vi "Logging Message Loop.vi"(8 "error in (no error)":cluster{"状态":bool, "代码":i32, "源":string} caption="错误输入（无错误）", 10 "数据队列":refnum<queue>, 11 "消息队列":T1) -> (0 "error out":cluster{"状态":bool, "代码":i32, "源":string} caption="错误输出")   [LabVIEW 2018, in "Logging.lvlib"]
doc: "消息循环子VI负责处理与记录数据相关的消息。"
uses:
  Logging.lvlib
  support/Message Queue/All Message Queues.ctl
  support/Message Queue/Message Cluster.ctl
  Logging Configuration.ctl
  Logging State.ctl
  support/Message Queue/Enqueue Message (Single).vi
  <vilib>/Utility/error.llb/Error Cluster From Error Code.vi
  <vilib>/ErrorRing/Error Ring.xnode
  support/Message Queue/Message Queue.lvlib
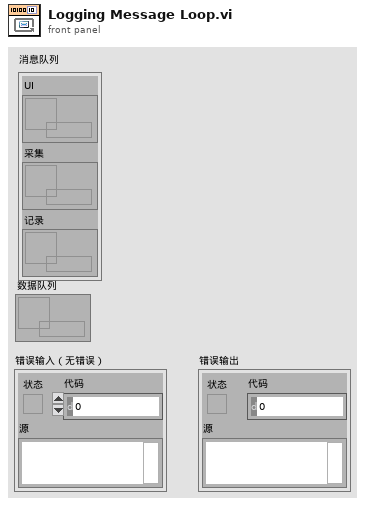
[diagram p1: front panel]
types:
  T1 = typedef "Message Queue.lvlib/All Message Queues.ctl" = cluster{"UI":refnum<queue>, "采集":refnum<queue>, "记录":refnum<queue>}
  T2 = typedef "Logging.lvlib/Logging Configuration.ctl" = cluster{"记录文件基路径":path, "TDMS文件引用":refnum<k34>}
  T3 = typedef "Logging.lvlib/Logging State.ctl" = enum16{"Idle", "Logging"}
  T4 = enum16{"open", "open or create", "create or replace", "create", "open (read-only)"}
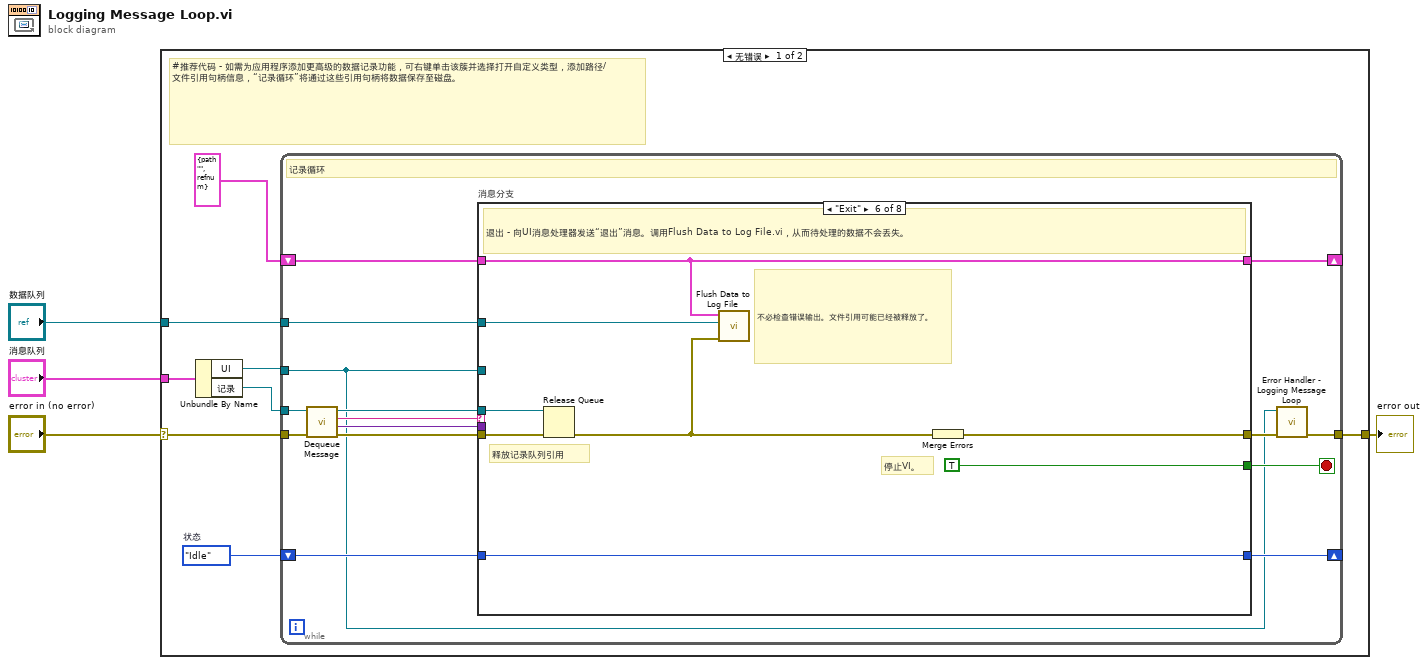
[diagram p0: block diagram]
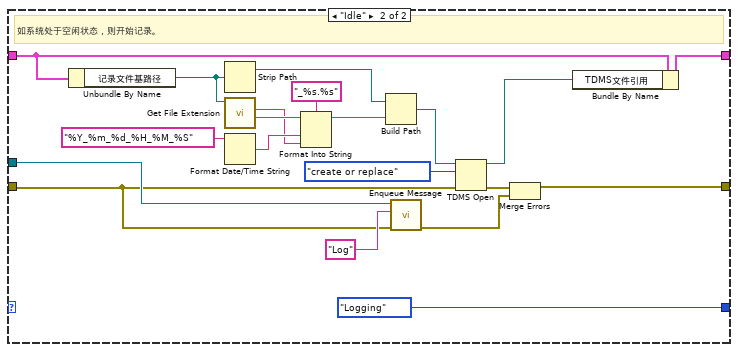
[diagram p4: hidden frame]
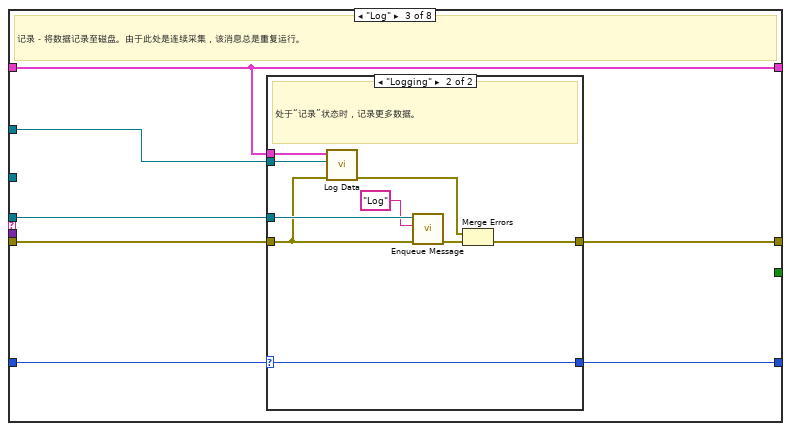
[diagram p5: hidden frame]
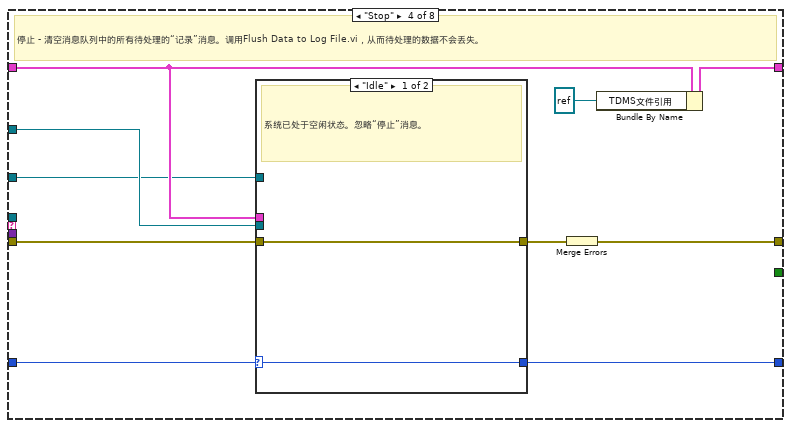
[diagram p7: hidden frame]
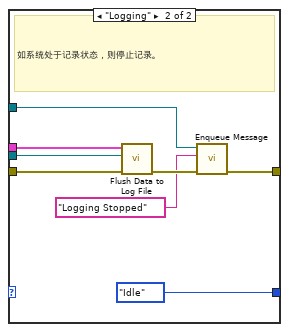
[diagram p8: hidden frame]
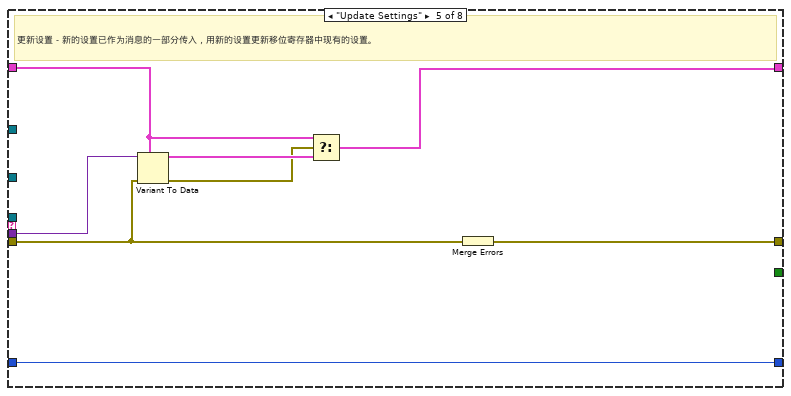
[diagram p9: hidden frame]
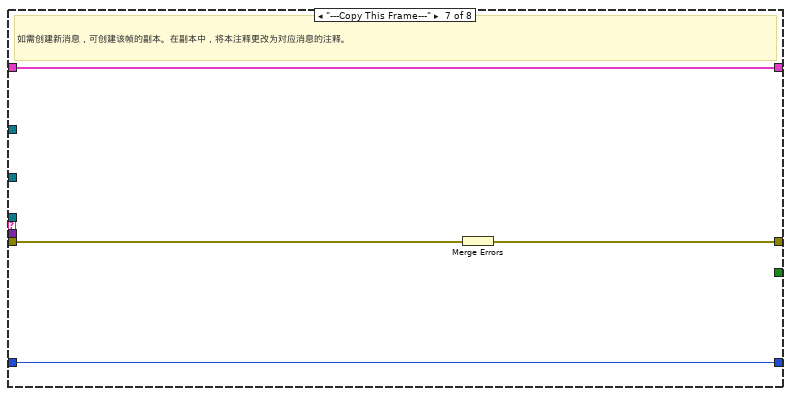
[diagram p10: hidden frame]
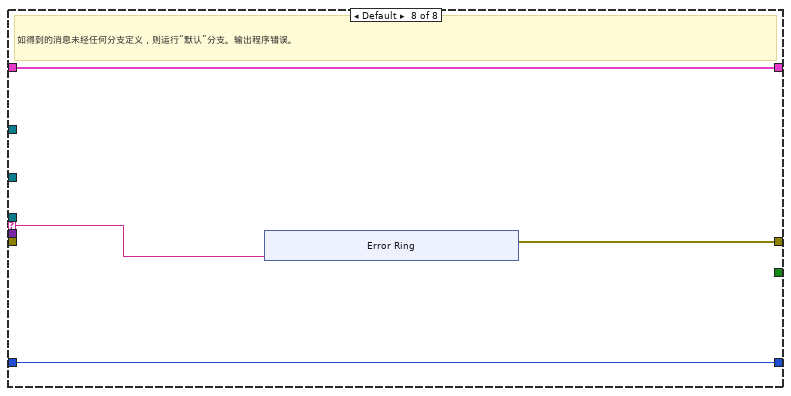
[diagram p11: hidden frame]
diagram:
  n1 = case shown="无错误" "error in (no error)" {
    selector: "error in (no error)" -> [w8 w130]
    tunnel: "消息队列" -> [w12 _]
    tunnel: [w10 w130] -> w3
    tunnel: "数据队列" -> [w7 _]
    frame No Error {
      w5 = Logging_State."Idle"  # 状态
      # "#推荐代码 - 如需为应用程序添加更高级的数据记录功能，可右键单击该簇并选择打开自定义类型，添加路径/文件引用句柄信息，“记录循环”将通过这些引用句柄将数据保存至磁盘。"
      n2 = Unbundle By Name(w12) -> ("UI"=w6:refnum<queue>, "记录"=w11:refnum<queue>)
      n3 = while {
        tunnel: w11 -> [w19]
        shift-right: [w26] -> _
        shift-left: T2 {"记录文件基路径"=path "", "TDMS文件引用"=refnum} ("Logging Configuration") -> [w27]
        tunnel: w6 -> [w13]
        tunnel: w7 -> [w18]
        shift-right: [w16] -> _
        shift-left: w5 -> [w17]
        tunnel: w8 -> [w24]
        tunnel: [w15] -> w10
        stop <- w25 stop-if-true
        # "记录循环"
        n4 = call "Dequeue Message.vi"("error in (no error)"=w24, "消息队列"=w19) -> ("error out"=w23:cluster{"状态":bool, "代码":i32, "源":string}, "消息数据"=w21:variant, "消息"=w22:string, "消息队列副本"=w20:refnum<queue>)  [unwired: 6 in]
        n5 = case "消息分支" shown="\"Exit\"" w22 {
          selector: w22 -> [_ _ _ _ _ _ _ w119]
          tunnel: w20 -> [_ w36 w66 _ _ w111 _ _]
          tunnel: w23 -> [w29 w35 w64 w82 w100 w112 w118 _]
          tunnel: [w29 w37 w67 w88 w106 w113 w116 w120] -> w14
          tunnel: w27 -> [w30 w34 w63 w83 w104 w109 w117 w122]
          tunnel: [w30 w33 w63 w86 w101 w109 w117 w122] -> w26
          tunnel: [_ _ _ _ _ TRUE _ _] -> w25
          tunnel: w21 -> [_ _ _ _ w105 _ _ _]
          tunnel: w13 -> [_ _ _ w79 _ _ _ _]
          tunnel: w18 -> [_ _ w65 w84 _ w108 _ _]
          tunnel: w17 -> [w28 w32 w62 w81 w99 w107 w115 w121]
          tunnel: [w28 w31 w61 w80 w99 w107 w115 w121] -> w16
          frame "Initialize" {
            # "初始化－第一次启动时将被调用。当前不包含任何操作。"
          }
          frame "Start" {
            # "开始 - 发送“记录”消息，开始记录。根据记录文件基路径的值生成一个唯一的带时间标识的TDMS文件名。"
            n6 = case shown="\"Logging\"" w32 {
              selector: w32 -> [w39 _]
              tunnel: [w38 w42] -> w37
              tunnel: w36 -> [_ w43]
              tunnel: w35 -> [w38 w41]
              tunnel: w34 -> [w40 w44]
              tunnel: [w40 w46] -> w33
              tunnel: [w39 Logging_State."Logging" ("State")] -> w31
              frame "Logging" {
                # "系统已处于记录状态。忽略“开始”消息。"
              }
              frame "Idle" {
                # "如系统处于空闲状态，则开始记录。"
                n7 = Unbundle By Name(w44) -> ("记录文件基路径"=w59:path)
                n8 = Strip Path(path=w59) -> (stripped path=w56:path)  [unwired: 1 out]
                n9 = call <vilib>:"Get File Extension.vi"("file"=w59) -> ("filename without extension"=w57:string, "lowercase file extension"=w53:string)  [unwired: 6 in, 3 out]
                n10 = Format Date/Time String(time format string (%c)="%Y_%m_%d_%H_%M_%S") -> (date/time string=w54:string)  [unwired: 2 in]
                n11 = Format Into String(format string="_%s.%s", initial string=w57, w54, w53) -> (resulting string=w52:string)  [unwired: 1 in, 1 out]
                n12 = Build Path(base path=w56, name or relative path=w52) -> (appended path=w51:path)
                n13 = call-poly "Enqueue Message.vi"("error in (no error)"=w41, "消息"="Log" ("Message"), "消息队列"=w43) -> ("error out"=w49:cluster{"状态":bool, "代码":i32, "源":string})  [unwired: 7 in, 1 out]
                n14 = TDMS Open(8:w41, 10:T4."create or replace" ("operation (0:open)"), 11:w51) -> (0:w50:errorcluster, 3:w47:refnum<k34>)  [unwired: 4 in]
                n15 = Merge Errors(w50, w49) -> (w42:errorcluster)
                n16 = Bundle By Name(cluster=w44, "TDMS文件引用"=w47) -> (w46:T2)
              }
            }
          }
          frame "Log" {
            # "记录－将数据记录至磁盘。由于此处是连续采集，该消息总是重复运行。"
            n17 = case shown="\"Logging\"" w62 {
              selector: w62 -> [w69 w71]
              tunnel: [w68 w78] -> w67
              tunnel: w66 -> [_ w76]
              tunnel: w65 -> [_ w75]
              tunnel: w64 -> [w68 w70]
              tunnel: w63 -> [_ w72]
              tunnel: [w69 w71] -> w61
              frame "Idle" {
                # "如记录处于空闲状态，则忽略“记录”消息。"
              }
              frame "Logging" {
                # "处于“记录”状态时，记录更多数据。"
                n18 = call "Log Data.vi"("error in (no error)"=w70, "数据队列"=w75, "记录配置"=w72) -> ("error out"=w74:cluster{"状态":bool, "代码":i32, "源":string})  [unwired: 8 in]
                n19 = call-poly "Enqueue Message.vi"("error in (no error)"=w70, "消息"="Log" ("Message"), "消息队列"=w76) -> ("error out"=w77:cluster{"状态":bool, "代码":i32, "源":string})  [unwired: 7 in, 1 out]
                n20 = Merge Errors(w74, w77) -> (w78:errorcluster)
              }
            }
          }
          frame "Stop" {
            # "停止 - 清空消息队列中的所有待处理的“记录”消息。调用Flush Data to Log File.vi，从而待处理的数据不会丢失。"
            n21 = case shown="\"Idle\"" w81 {
              selector: w81 -> [w89 _]
              tunnel: [w90 w93] -> w87
              tunnel: w84 -> [_ w97]
              tunnel: w83 -> [_ w96]
              tunnel: w82 -> [w90 w95]
              tunnel: [w89 Logging_State."Idle" ("State")] -> w80
              tunnel: w79 -> [_ w92]
              frame "Idle" {
                # "系统已处于空闲状态。忽略“停止”消息。"
              }
              frame "Logging" {
                # "如系统处于记录状态，则停止记录。"
                n22 = call "Flush Data to Log File.vi"("error in (no error)"=w95, "数据队列"=w97, "记录配置"=w96) -> ("error out"=w98:cluster{"状态":bool, "代码":i32, "源":string})  [unwired: 8 in]
                n23 = call-poly "Enqueue Message.vi"("error in (no error)"=w98, "消息"="Logging Stopped", "消息队列"=w92) -> ("error out"=w93:cluster{"状态":bool, "代码":i32, "源":string})  [unwired: 7 in, 1 out]
              }
            }
            n24 = Merge Errors(w87) -> (w88:errorcluster)
            n25 = Bundle By Name(cluster=w83, "TDMS文件引用"=refnum<k34> refnum ("TDMS File Reference")) -> (w86:T2)
          }
          frame "Update Settings" {
            # "更新设置－新的设置已作为消息的一部分传入，用新的设置更新移位寄存器中现有的设置。"
            n26 = Variant To Data(error in=w100, type=w104, Variant=w105) -> (data=w103:T2, error out=w102:errorcluster)
            n27 = Select(t=w104, s=w102, f=w103) -> (s? t:f=w101:T2)
            n28 = Merge Errors(w100) -> (w106:errorcluster)
          }
          frame "Exit" {
            # "不必检查错误输出。文件引用可能已经被释放了。"
            # "释放记录队列引用"
            # "停止VI。"
            # "退出 - 向UI消息处理器发送“退出”消息。调用Flush Data to Log File.vi，从而待处理的数据不会丢失。"
            n29 = Release Queue(queue=w111, error in (no error)=w112) -> (error out=w110:errorcluster)  [unwired: 1 in, 2 out]
            n30 = call "Flush Data to Log File.vi"("error in (no error)"=w110, "数据队列"=w108, "记录配置"=w109) -> ()  [unwired: 8 in, 1 out]
            n31 = Merge Errors(w110) -> (w113:errorcluster)
          }
          frame "---Copy This Frame---" {
            # "如需创建新消息，可创建该帧的副本。在副本中，将本注释更改为对应消息的注释。"
            n32 = Merge Errors(w118) -> (w116:errorcluster)
          }
          frame Default {
            # "如得到的消息未经任何分支定义，则运行“默认”分支。输出程序错误。"
            n33 = xnode ("Error Ring")("参数 0"=w119) -> ("错误输出"=w120:errorcluster)
          }
        }
        n34 = call "Error Handler - Logging Message Loop.vi"("error in (no error)"=w14, "消息队列"=w13) -> ("错误输入副本"=w15:cluster{"状态":bool, "代码":i32, "源":string})  [unwired: 8 in, 1 out]
      }
    }
    frame Error {
    }
  }
  "error out" <- w3
